vi "ForthCode.vi"() -> ()   [LabVIEW 2018]
panel:
  in  "String":string
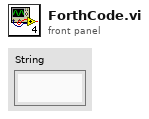
[diagram p1: front panel]
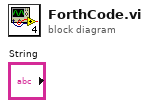
[diagram p0: block diagram]
diagram:
